vi "quiz3_vale.vi"() -> ()   [LabVIEW 2017]
panel:
  out "Usuarios Existentes 2":string[][](array[string])
  out "Leer 2":string[][](array[string])
  out "array 2":string[][](array[string])
  out "Tamaño users 2":i32
  out "Tab Control 2":enum32{"Page 1", "Page 2", "Page 3"}(tab)
  in  "Ingresar 2":bool
  in  "Usuario 2":string
  in  "Contraseña  2":string
  in  "Regresar 3":bool
  in  "ver usuarios 2":bool
  in  "Borrar usuario 2":string
  in  "Eliminar 2":bool
  in  "Agregar 2":bool
  in  "Contraseña usuario 2":string
  in  "nuevo usuario 2":string
  in  "Regresar 4":bool
  out "Leer":string[][](array[string])
  out "Usuarios Existentes":string[][](array[string])
  out "Tamaño users":i32
  out "array":string[][](array[string])
  out "Tab Control":enum32{"Page 1", "Page 2", "Page 3"}(tab)
  in  "Ingresar":bool
  in  "Usuario":string
  in  "Contraseña":string
  in  "Regresar":bool
  in  "ver usuarios":bool
  in  "Borrar usuario":string
  in  "Eliminar":bool
  in  "Agregar":bool
  in  "Contraseña usuario":string
  in  "nuevo usuario":string
  in  "Regresar 2":bool
  # "HOLIII..!"
  # "HOLIII..!"
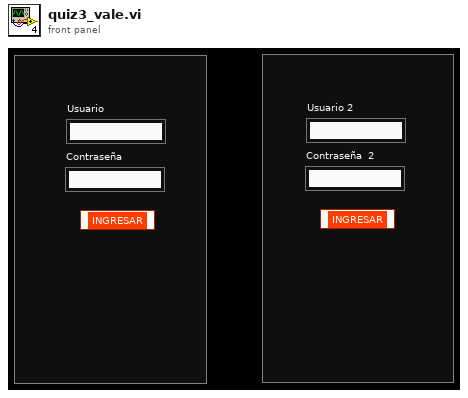
[diagram p1: front panel]
types:
  T1 = enum16{"open", "replace", "create", "open or create", "replace or create", "replace or create with confirmation"}
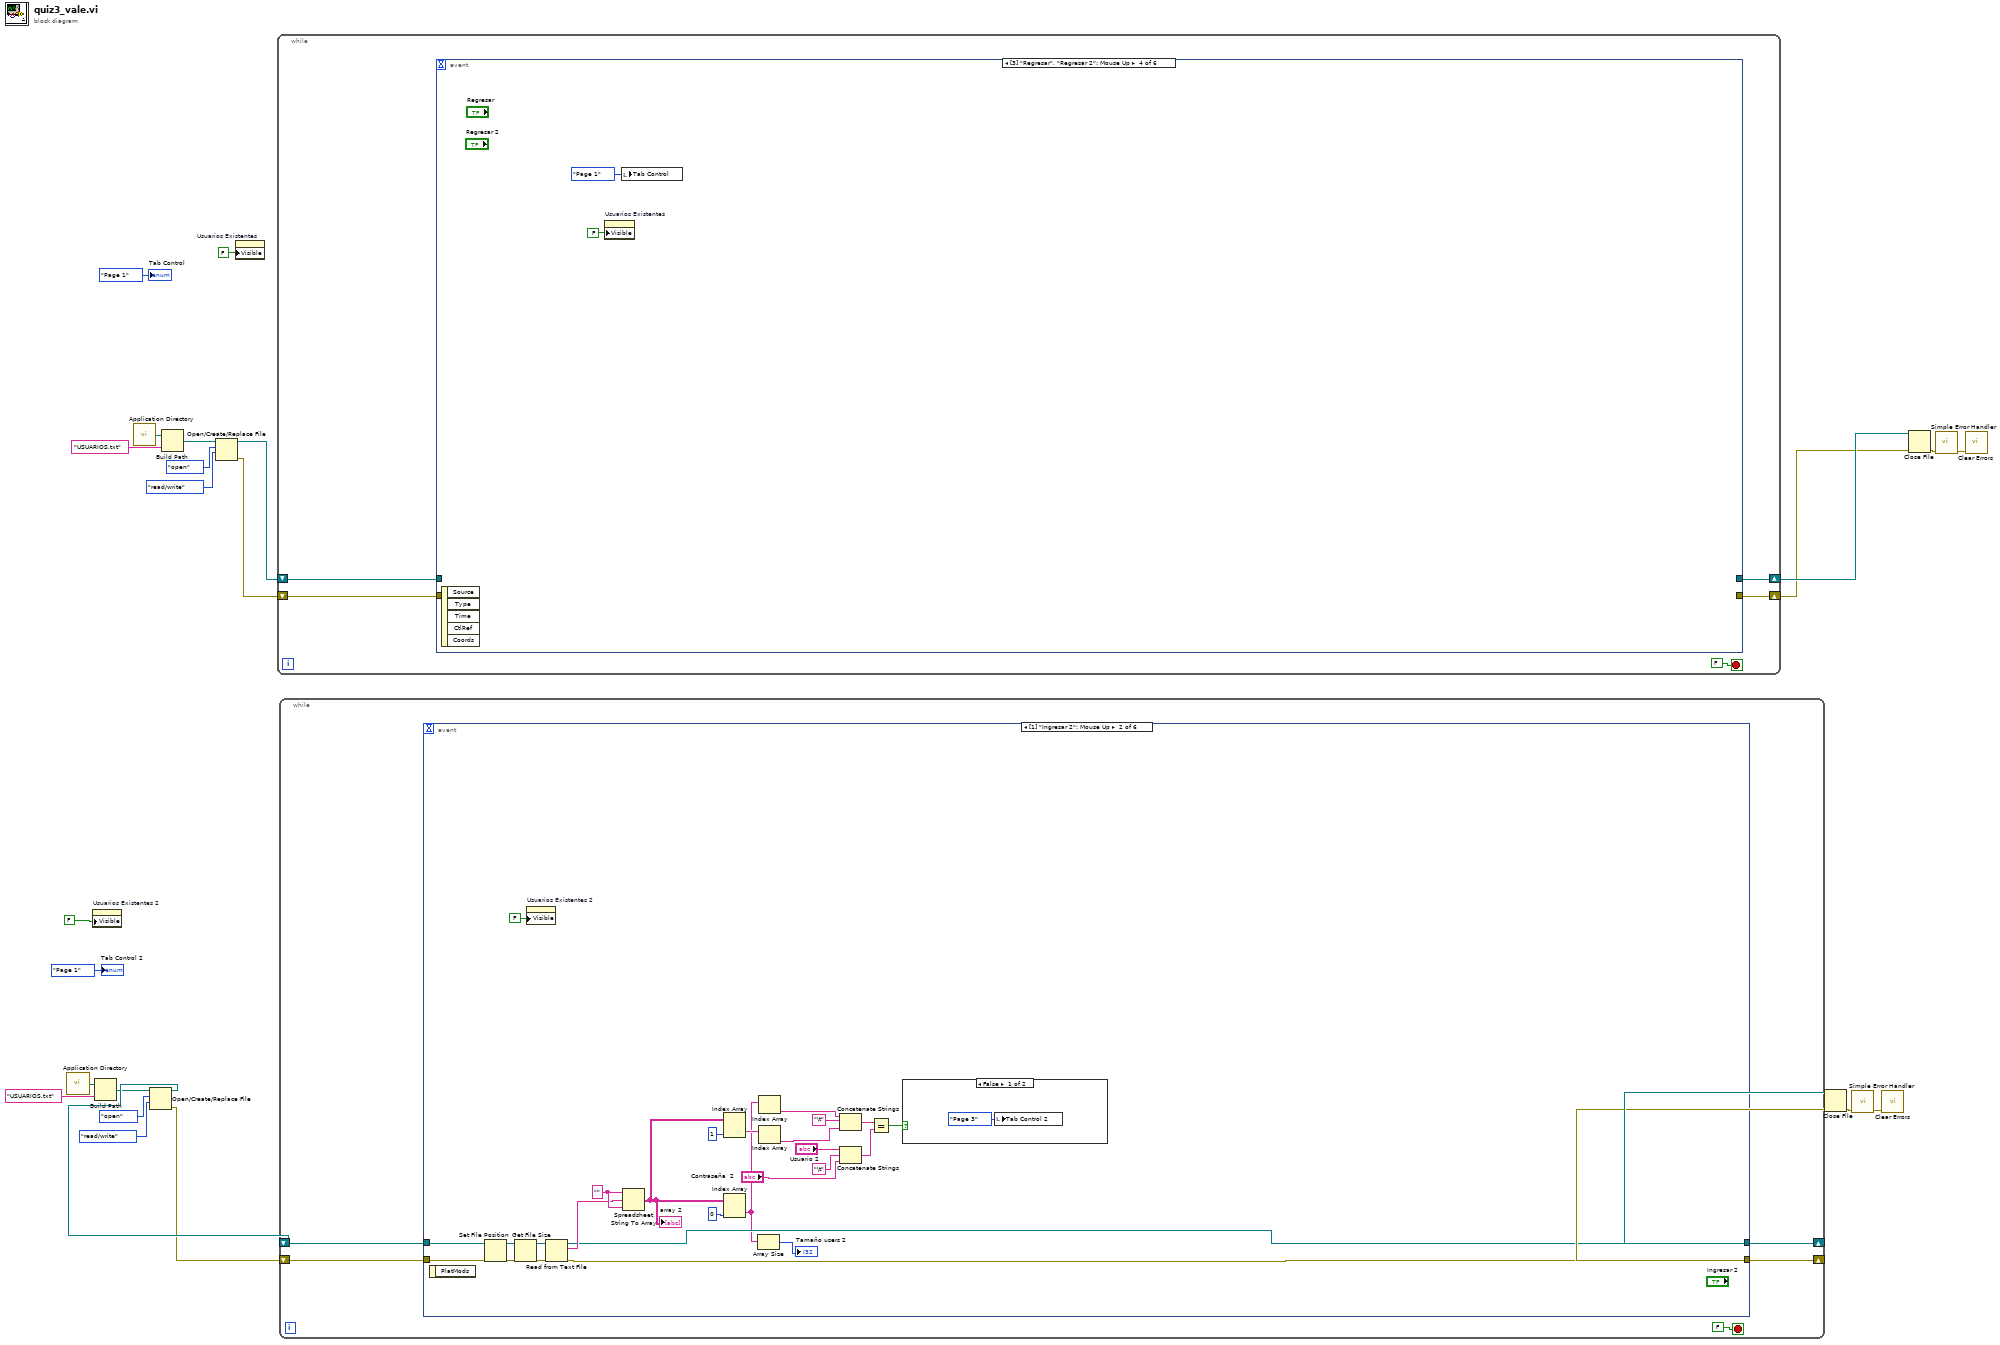
[diagram p0: block diagram]
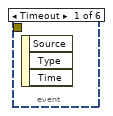
[diagram p2: hidden frame]
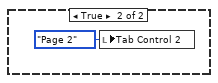
[diagram p3: hidden frame]
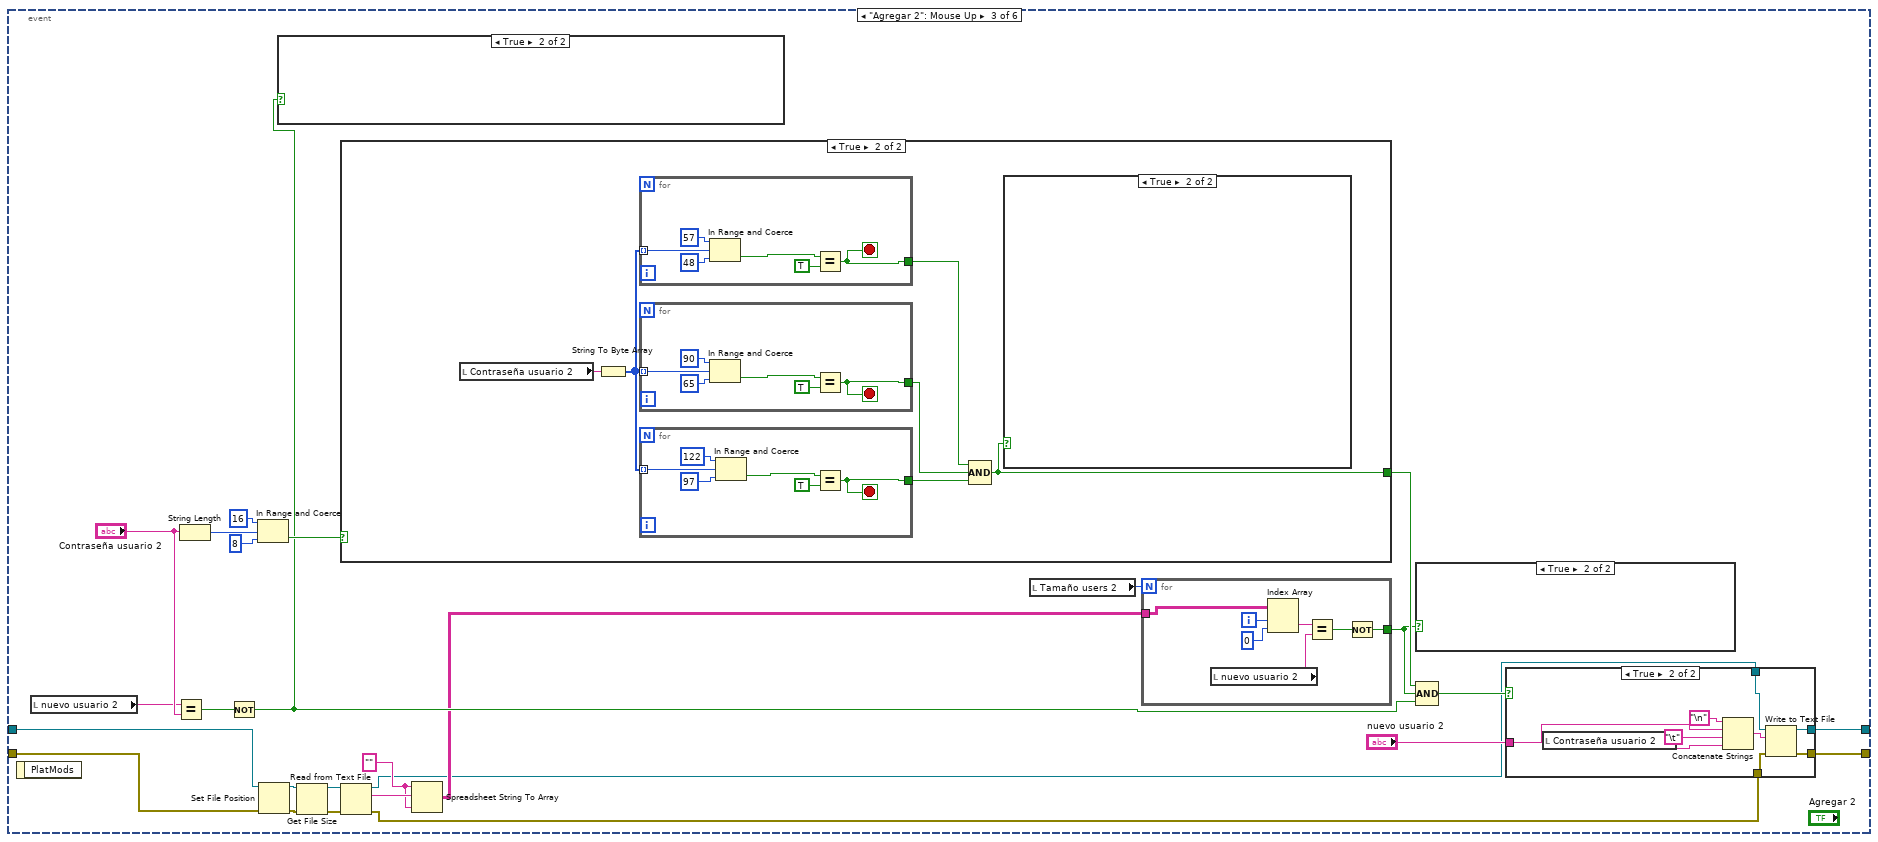
[diagram p4: hidden frame]
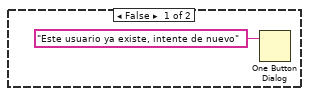
[diagram p5: hidden frame]
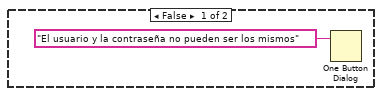
[diagram p6: hidden frame]
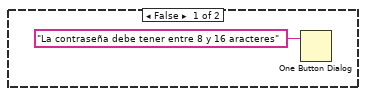
[diagram p8: hidden frame]
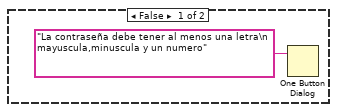
[diagram p9: hidden frame]
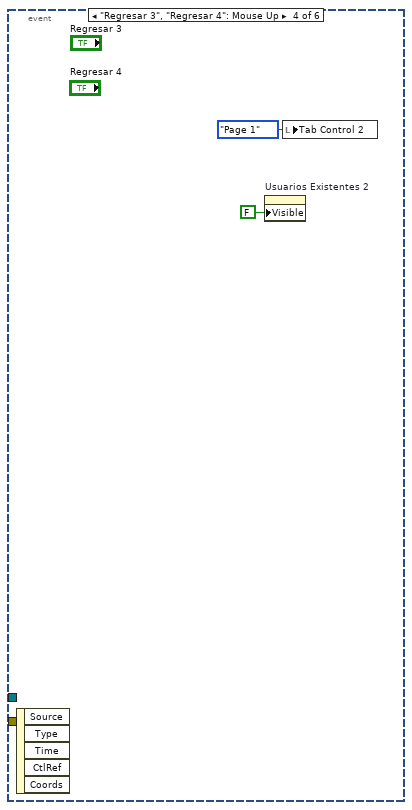
[diagram p10: hidden frame]
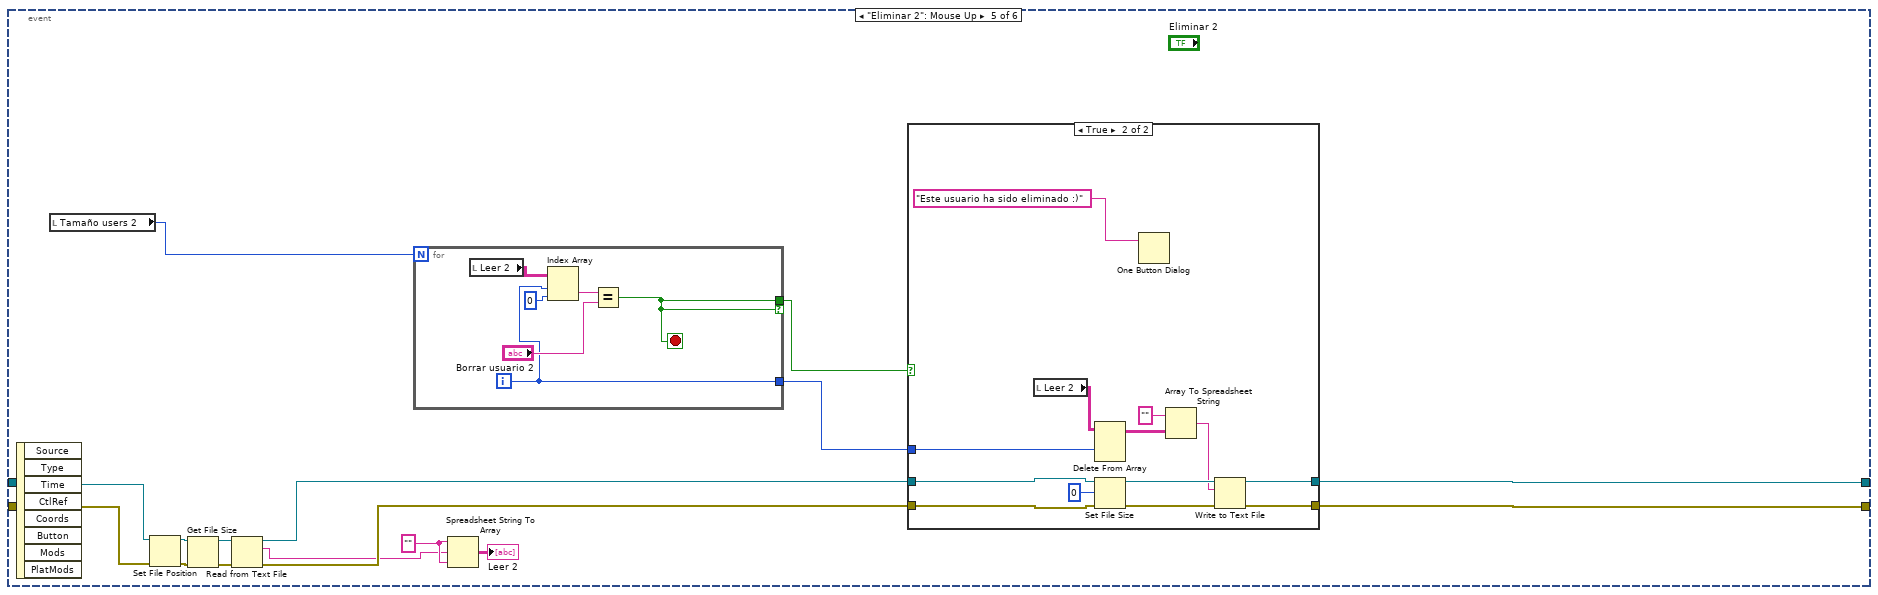
[diagram p11: hidden frame]
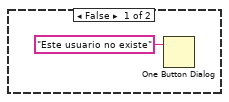
[diagram p12: hidden frame]
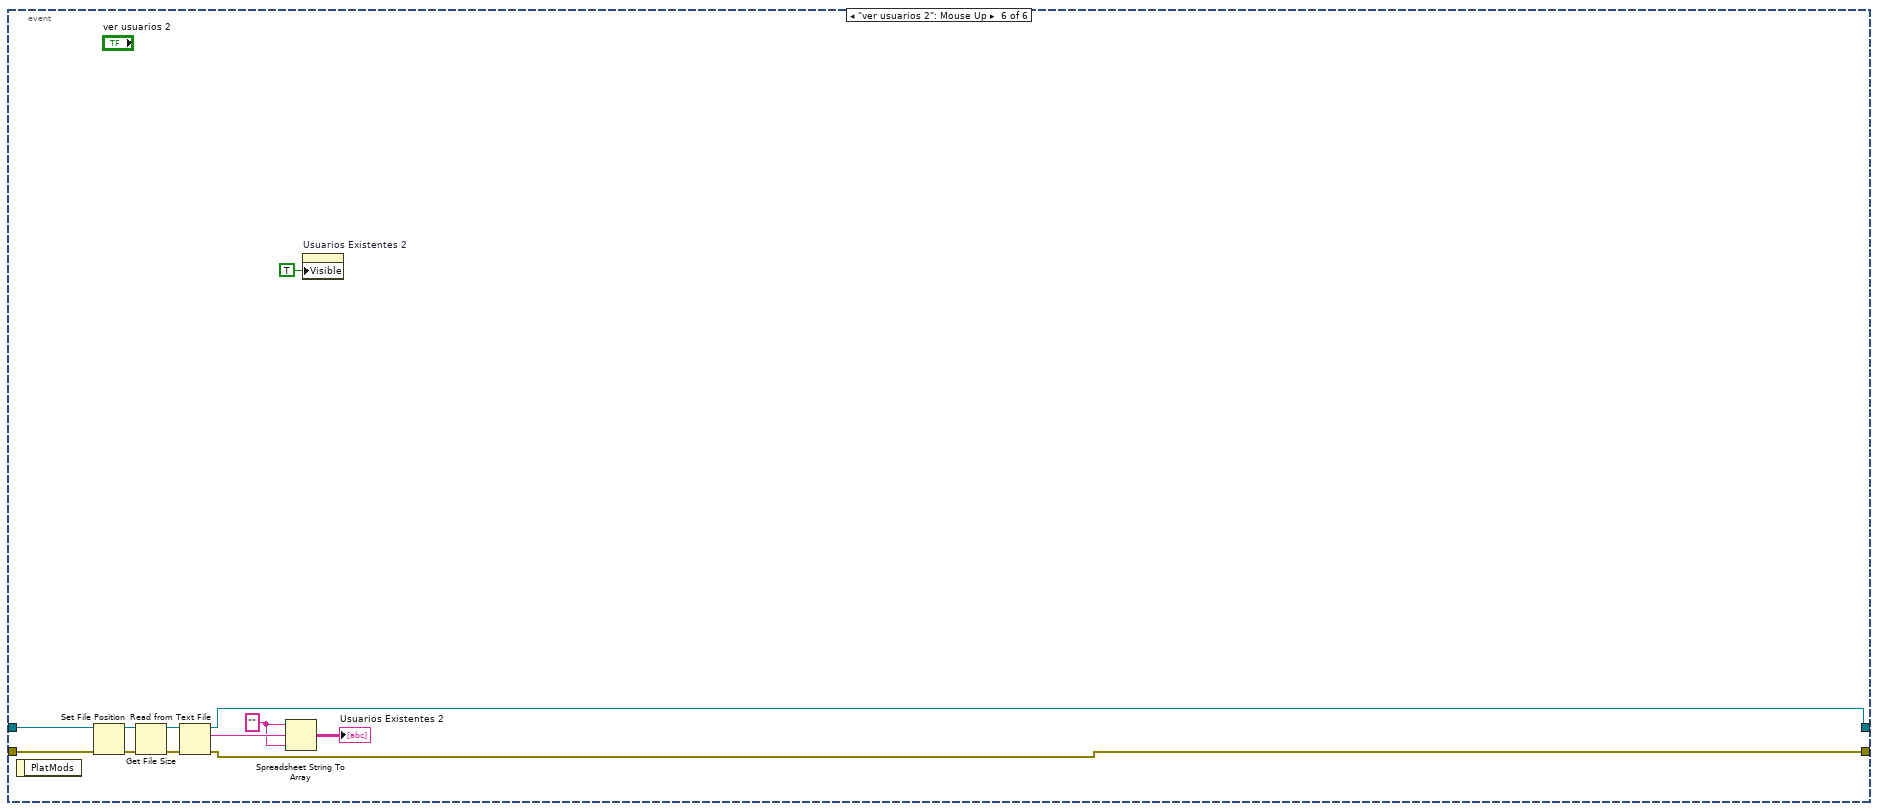
[diagram p13: hidden frame]
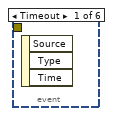
[diagram p14: hidden frame]
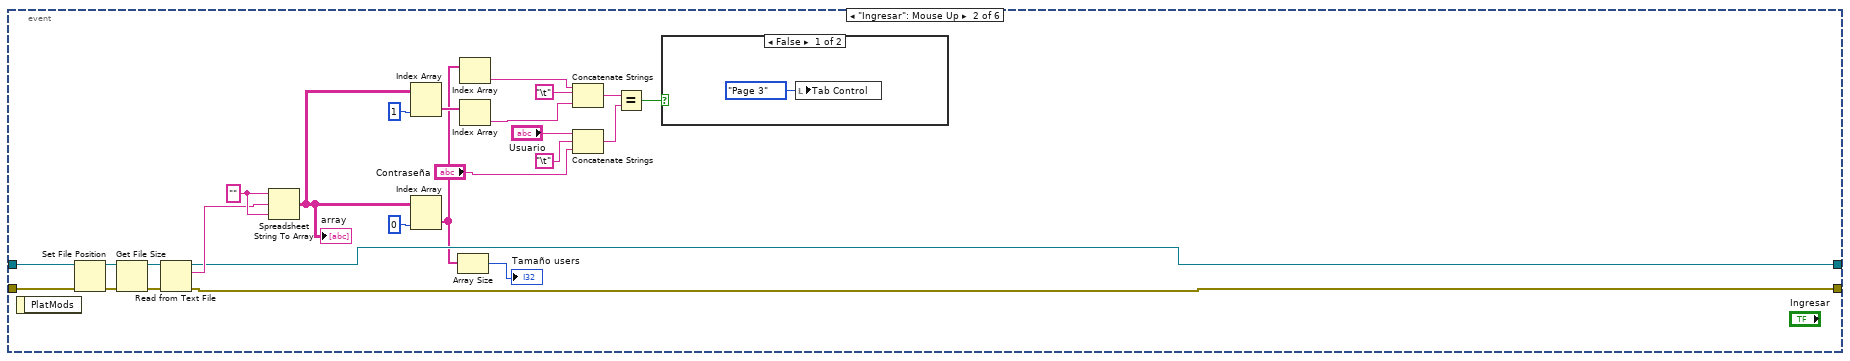
[diagram p15: hidden frame]
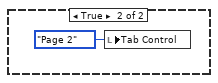
[diagram p16: hidden frame]
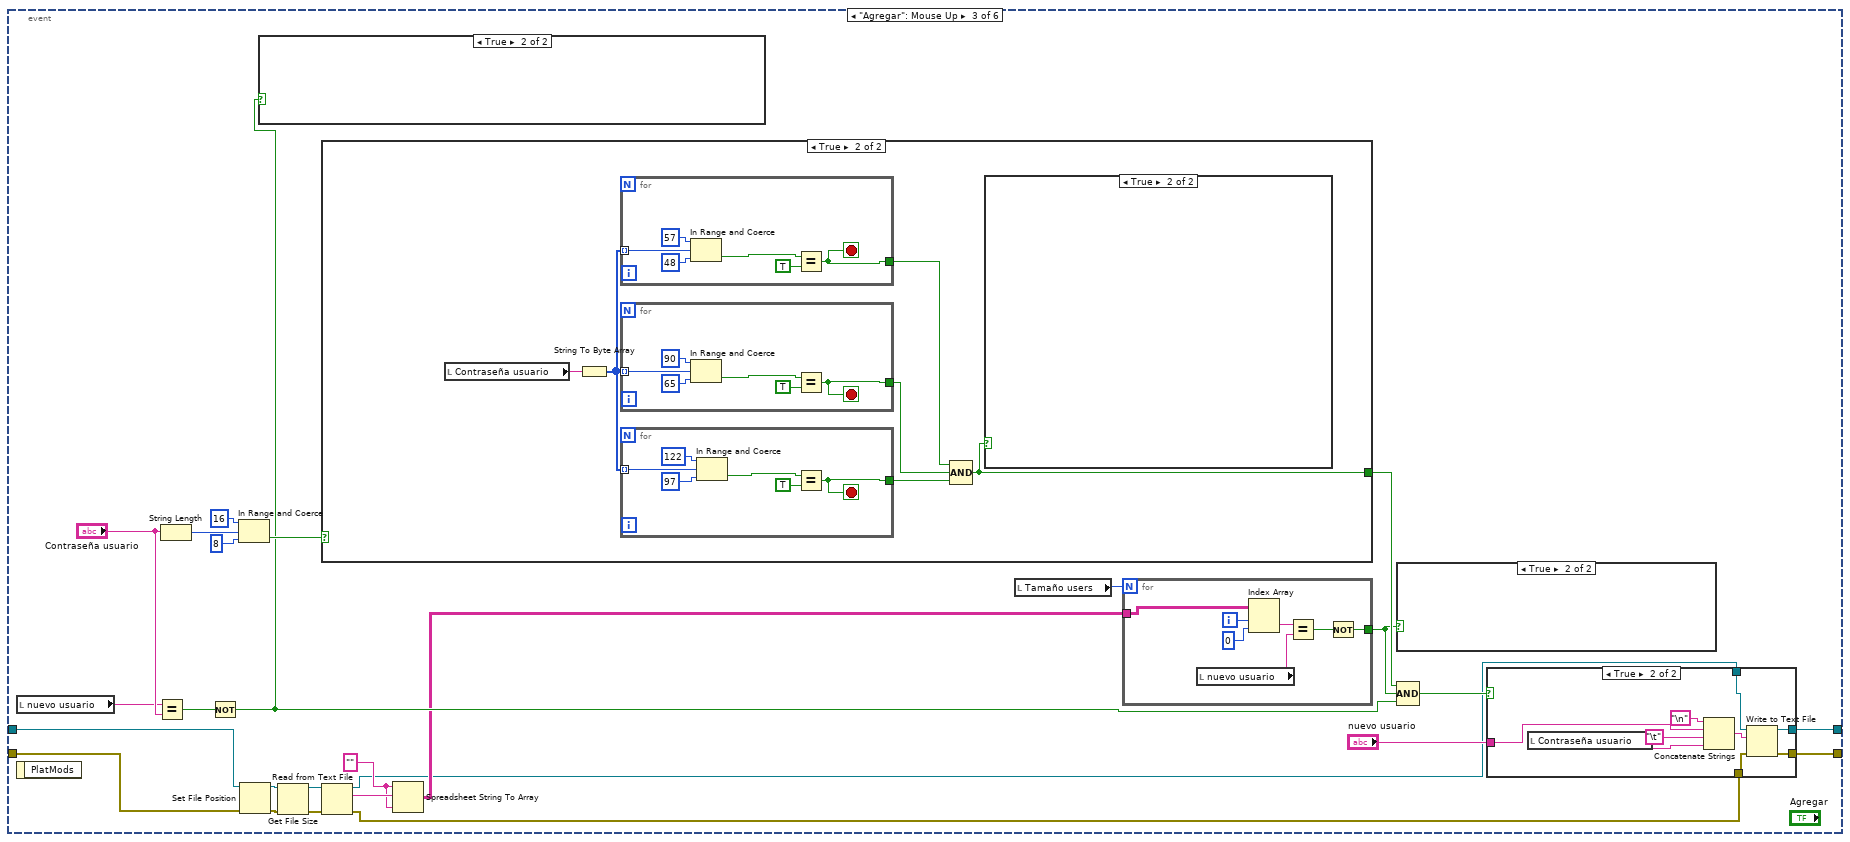
[diagram p17: hidden frame]
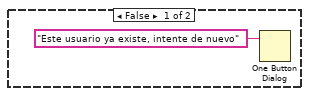
[diagram p18: hidden frame]
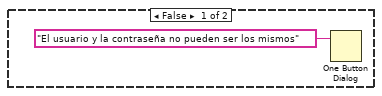
[diagram p19: hidden frame]
diagram:
  n1 = call <vilib>:"Application Directory.vi"() -> ("Application Directory"=w11:path)
  n2 = property on="Usuarios Existentes 2" class="Arr (strict)"("Visible"=FALSE) -> ()  [unwired: 2 in, 2 out]
  n3 = Build Path(base path=w11, name or relative path="USUARIOS.txt") -> (appended path=w10:path)
  n4 = call <vilib>:"Application Directory.vi"() -> ("Application Directory"=w24:path)
  n5 = Open/Create/Replace File(file path (use dialog)=w10, operation (0:open)=T1."open", access (0:read/write)=enum16{"read/write", "read-only", "write-only"}."read/write") -> (refnum out=w14:refnum<file>, error out=w13:errorcluster)  [unwired: 3 in, 1 out]
  n6 = Build Path(base path=w24, name or relative path="USUARIOS.txt") -> (appended path=w23:path)
  n7 = Open/Create/Replace File(file path (use dialog)=w23, operation (0:open)=T1."open", access (0:read/write)=enum16{"read/write", "read-only", "write-only"}."read/write") -> (refnum out=w26:refnum<file>, error out=w1:errorcluster)  [unwired: 3 in, 1 out]
  n8 = property on="Usuarios Existentes" class="Arr (strict)"("Visible"=FALSE) -> ()  [unwired: 2 in, 2 out]
  n9 = while {
    shift-right: [w28] -> w20
    shift-left: w26 -> [w30]
    shift-right: [w29] -> w19
    shift-left: w1 -> [w27]
    stop <- FALSE stop-if-true
    n10 = event shown="[3] \"Regresar\", \"Regresar 2\": Mouse Up" {
      selector: _ -> [_ _ _ _ _ _]
      dyn-events: _ -> [_ _ _ _ _ _]
      timeout: _ -> [_ _ _ _ _ _]
      tunnel: w27 -> [_ w56 w65 _ w136 w171]
      tunnel: w30 -> [_ w53 w64 _ w137 w172]
      tunnel: [_ w42 w78 _ w142 w166] -> w28
      tunnel: [_ w41 w79 _ w143 w167] -> w29
      event Timeout {
        n11 = event-data() -> ()  [unwired: 1 in, 3 out]
      }
      event "Ingresar": Mouse Up {
        w45 = "" ("format string")
        n12 = event-data() -> ()  [unwired: 1 in, 1 out]
        n13 = Set File Position(refnum=w53, error in=w56) -> (refnum out=w52:refnum<file>, error out=w55:errorcluster)  [unwired: 2 in]
        n14 = Get File Size(file=w52, error in=w55) -> (refnum out=w51:refnum<file>, 0:w54:errorcluster)  [unwired: 1 out]
        n15 = Read from Text File(file (use dialog)=w51, error in=w54) -> (refnum out=w42:refnum<file>, text=w44:string, error out=w41:errorcluster)  [unwired: 2 in, 1 out]
        n16 = Spreadsheet String To Array(format string=w45, spreadsheet string=w44, array type (2D Dbl)=w45) -> (array=w38:string[][])  [unwired: 1 in]
        "array" <- w38
        n17 = Index Array(array=w38, index (col)=1 ("disabled index (col)")) -> (element=w43:string[])  [unwired: 1 in]
        n18 = Index Array(array=w38, index (col)=0 ("disabled index (col)")) -> (element=w37:string[])  [unwired: 1 in]
        n19 = Array Size(array=w37) -> (size(s)=→"Tamaño users":i32)
        n20 = Index Array(array=w37) -> (element=w32:string)  [unwired: 1 in]
        n21 = Index Array(array=w43) -> (element=w33:string)  [unwired: 1 in]
        n22 = Concatenate Strings(w32, "\t", w33) -> (w40:string)
        n23 = Concatenate Strings("Usuario", "\t", "Contraseña") -> (w39:string)
        n24 = Equal?(x=w40, y=w39) -> (x = y?=w35:bool)
        n25 = case shown="False" w35 {
          frame False {
            n26 = local write "Tab Control"(enum32{"Page 1", "Page 2", "Page 3"}."Page 3" ("Tab Control")) -> ()
          }
          frame True {
            n27 = local write "Tab Control"(enum32{"Page 1", "Page 2", "Page 3"}."Page 2" ("Tab Control")) -> ()
          }
        }
      }
      event "Agregar": Mouse Up {
        w62 = "" ("format string")
        n28 = local read "nuevo usuario"() -> (w72:string)
        n29 = event-data() -> ()  [unwired: 1 in, 1 out]
        n30 = Equal?(x=w72, y="Contraseña usuario") -> (x = y?=w74:bool)
        n31 = String Length(string="Contraseña usuario") -> (length=w84:i32)
        n32 = Not(x=w74) -> (.not. x?=w73:bool)
        n33 = In Range and Coerce(upper limit=16, x=w84, lower limit=8) -> (In Range?=w81:bool)  [unwired: 1 out]
        n34 = Set File Position(refnum=w64, error in=w65) -> (refnum out=w68:refnum<file>, error out=w66:errorcluster)  [unwired: 2 in]
        n35 = case shown="True" w73 {
          frame False {
            n36 = One Button Dialog(message="El usuario y la contraseña no pueden ser los mismos") -> ()  [unwired: 1 in, 1 out]
          }
          frame True {
          }
        }
        n37 = Get File Size(file=w68, error in=w66) -> (refnum out=w69:refnum<file>, 0:w67:errorcluster)  [unwired: 1 out]
        n38 = case shown="True" w81 {
          tunnel: [_ w104] -> w75
          frame False {
            n39 = One Button Dialog(message="La contraseña debe tener entre 8 y 16 aracteres") -> ()  [unwired: 1 in, 1 out]
          }
          frame True {
            n40 = local read "Contraseña usuario"() -> (w109:string)
            n41 = String To Byte Array(string=w109) -> (unsigned byte array=w107:u8[])
            n42 = for {
              tunnel: w107 -> [w117] mode=indexing
              tunnel: [w116] -> w108
              stop <- w116 stop-if-true
              n43 = In Range and Coerce(upper limit=u8 57, x=w117, lower limit=u8 48) -> (In Range?=w119:bool)  [unwired: 1 out]
              n44 = Equal?(x=w119, y=TRUE) -> (x = y?=w116:bool)
            }
            n45 = for {
              tunnel: w107 -> [w113] mode=indexing
              tunnel: [w110] -> w106
              stop <- w110 stop-if-true
              n46 = In Range and Coerce(upper limit=u8 90, x=w113, lower limit=u8 65) -> (In Range?=w112:bool)  [unwired: 1 out]
              n47 = Equal?(x=w112, y=TRUE) -> (x = y?=w110:bool)
            }
            n48 = for {
              tunnel: w107 -> [w123] mode=indexing
              tunnel: [w124] -> w105
              stop <- w124 stop-if-true
              n49 = In Range and Coerce(upper limit=u8 122, x=w123, lower limit=u8 97) -> (In Range?=w126:bool)  [unwired: 1 out]
              n50 = Equal?(x=w126, y=TRUE) -> (x = y?=w124:bool)
            }
            n51 = Compound Arithmetic op=AND(w108, w106, w105) -> (w104:bool)
            n52 = case shown="True" w104 {
              frame False {
                n53 = One Button Dialog(message="La contraseña debe tener al menos una letra\n mayuscula,minuscula y un numero") -> ()  [unwired: 1 in, 1 out]
              }
              frame True {
              }
            }
          }
        }
        n54 = Read from Text File(file (use dialog)=w69, error in=w67) -> (refnum out=w59:refnum<file>, text=w63:string, error out=w60:errorcluster)  [unwired: 2 in, 1 out]
        n55 = Spreadsheet String To Array(format string=w62, spreadsheet string=w63, array type (2D Dbl)=w62) -> (array=w61:string[][])  [unwired: 1 in]
        n56 = local read "Tamaño users"() -> (w80:i32)
        n57 = for {
          N: w80 -> [_]
          tunnel: [w88] -> w70
          tunnel: w61 -> [w87]
          i -> [w92]
          n58 = local read "nuevo usuario"() -> (w90:string)
          n59 = Index Array(array=w87, index (row)=w92, index (col)=0 ("disabled index (col)")) -> (element=w91:string)
          n60 = Equal?(x=w91, y=w90) -> (x = y?=w89:bool)
          n61 = Not(x=w89) -> (.not. x?=w88:bool)
        }
        n62 = case shown="True" w70 {
          frame False {
            n63 = One Button Dialog(message="Este usuario ya existe, intente de nuevo") -> ()  [unwired: 1 in, 1 out]
          }
          frame True {
          }
        }
        n64 = Compound Arithmetic op=AND(w75, w70, w73) -> (w76:bool)
        n65 = case shown="True" w76 {
          tunnel: [_ w98] -> w78
          tunnel: [_ w97] -> w79
          tunnel: "nuevo usuario" -> [_ w96]
          tunnel: w59 -> [_ w95]
          tunnel: w60 -> [_ w94]
          frame False {
          }
          frame True {
            n66 = local read "Contraseña usuario"() -> (w99:string)
            n67 = Concatenate Strings("\n", w96, "\t", w99) -> (w100:string)
            n68 = Write to Text File(file (use dialog)=w95, text=w100, error in=w94) -> (refnum out=w98:refnum<file>, error out=w97:errorcluster)  [unwired: 1 in, 1 out]
          }
        }
      }
      event "Regresar", "Regresar 2": Mouse Up {
        n69 = event-data() -> ()  [unwired: 1 in, 5 out]
        n70 = property on="Usuarios Existentes" class="Arr (strict)"("Visible"=FALSE) -> ()  [unwired: 2 in, 2 out]
        n71 = local write "Tab Control"(enum32{"Page 1", "Page 2", "Page 3"}."Page 1" ("Tab Control")) -> ()
      }
      event "Eliminar": Mouse Up {
        w134 = "" ("format string")
        n72 = event-data() -> ()  [unwired: 1 in, 1 out]
        n73 = local read "Tamaño users"() -> (w145:i32)
        n74 = Set File Position(refnum=w137, error in=w136) -> (refnum out=w140:refnum<file>, error out=w138:errorcluster)  [unwired: 2 in]
        n75 = Get File Size(file=w140, error in=w138) -> (refnum out=w141:refnum<file>, 0:w139:errorcluster)  [unwired: 1 out]
        n76 = Read from Text File(file (use dialog)=w141, error in=w139) -> (refnum out=w135:refnum<file>, text=w133:string)  [unwired: 2 in, 2 out]
        n77 = for {
          N: w145 -> [_]
          tunnel: [w162] -> w144
          tunnel: [w159] -> w131 if=w159
          i -> [w162]
          stop <- w159 stop-if-true
          n78 = local read "Leer"() -> (w161:string[][])
          n79 = Index Array "Index Array"(array=w161, index (row)=w162, index (col)=0 ("disabled index (col)")) -> (element=w160:string)
          n80 = Equal?(x=w160, y="Borrar usuario") -> (x = y?=w159:bool)
        }
        n81 = Spreadsheet String To Array(format string=w134, spreadsheet string=w133, array type (2D Dbl)=w134) -> (array=→"Leer":string[][])  [unwired: 1 in]
        n82 = case shown="True" w131 {
          tunnel: w144 -> [_ w158]
          tunnel: w135 -> [_ w154]
          tunnel: [_ w152] -> w143
          tunnel: [_ w151] -> w142
          frame False {
            n83 = One Button Dialog(message="Este usuario no existe") -> ()  [unwired: 1 in, 1 out]
          }
          frame True {
            n84 = local read "Leer"() -> (w149:string[][])
            n85 = Delete From Array "Delete From Array"(array=w149, index (row)=w158) -> (array with subset deleted=w148:string[][])  [unwired: 2 in, 1 out]
            n86 = Set File Size(6:i64 0 ("size (in bytes)"), 7:w154) -> (0:w153:errorcluster, 3:w156:refnum<file>)  [unwired: 1 in]
            n87 = One Button Dialog(message="Este usuario ha sido eliminado :)") -> ()  [unwired: 1 in, 1 out]
            n88 = Array To Spreadsheet String(array=w148, 3:"" ("format string")) -> (spreadsheet string=w155:string)  [unwired: 1 in]
            n89 = Write to Text File(file (use dialog)=w156, text=w155, error in=w153) -> (refnum out=w151:refnum<file>, error out=w152:errorcluster)  [unwired: 1 in, 1 out]
          }
        }
      }
      event "ver usuarios": Mouse Up {
        w169 = "" ("format string")
        n90 = event-data() -> ()  [unwired: 1 in, 1 out]
        n91 = Set File Position(refnum=w172, error in=w171) -> (refnum out=w175:refnum<file>, error out=w173:errorcluster)  [unwired: 2 in]
        n92 = Get File Size(file=w175, error in=w173) -> (refnum out=w176:refnum<file>, 0:w174:errorcluster)  [unwired: 1 out]
        n93 = Read from Text File(file (use dialog)=w176, error in=w174) -> (refnum out=w166:refnum<file>, text=w170:string, error out=w167:errorcluster)  [unwired: 2 in, 1 out]
        n94 = Spreadsheet String To Array(format string=w169, spreadsheet string=w170, array type (2D Dbl)=w169) -> (array=→"Usuarios Existentes":string[][])  [unwired: 1 in]
        n95 = property on="Usuarios Existentes" class="Arr (strict)"("Visible"=TRUE) -> ()  [unwired: 2 in, 2 out]
      }
    }
  }
  n96 = while {
    shift-right: [w178] -> w7
    shift-left: w14 -> [w180]
    shift-right: [w179] -> w6
    shift-left: w13 -> [w177]
    stop <- FALSE stop-if-true
    n97 = event shown="[1] \"Ingresar 2\": Mouse Up" {
      selector: _ -> [_ _ _ _ _ _]
      dyn-events: _ -> [_ _ _ _ _ _]
      timeout: _ -> [_ _ _ _ _ _]
      tunnel: w177 -> [_ w207 w216 _ w288 w324]
      tunnel: w180 -> [_ w204 w215 _ w289 w325]
      tunnel: [_ w193 w229 _ w294 w319] -> w178
      tunnel: [_ w192 w230 _ w295 w320] -> w179
      event Timeout {
        n98 = event-data() -> ()  [unwired: 1 in, 3 out]
      }
      event "Ingresar 2": Mouse Up {
        w196 = "" ("format string")
        n99 = event-data() -> ()  [unwired: 1 in, 1 out]
        n100 = Set File Position(refnum=w204, error in=w207) -> (refnum out=w203:refnum<file>, error out=w206:errorcluster)  [unwired: 2 in]
        n101 = Get File Size(file=w203, error in=w206) -> (refnum out=w202:refnum<file>, 0:w205:errorcluster)  [unwired: 1 out]
        n102 = property on="Usuarios Existentes 2" class="Arr (strict)"("Visible"=FALSE) -> ()  [unwired: 2 in, 2 out]
        n103 = Read from Text File(file (use dialog)=w202, error in=w205) -> (refnum out=w193:refnum<file>, text=w195:string, error out=w192:errorcluster)  [unwired: 2 in, 1 out]
        n104 = Spreadsheet String To Array(format string=w196, spreadsheet string=w195, array type (2D Dbl)=w196) -> (array=w189:string[][])  [unwired: 1 in]
        "array 2" <- w189
        n105 = Index Array(array=w189, index (col)=1 ("disabled index (col)")) -> (element=w194:string[])  [unwired: 1 in]
        n106 = Index Array(array=w189, index (col)=0 ("disabled index (col)")) -> (element=w188:string[])  [unwired: 1 in]
        n107 = Array Size(array=w188) -> (size(s)=→"Tamaño users 2":i32)
        n108 = Index Array(array=w188) -> (element=w183:string)  [unwired: 1 in]
        n109 = Index Array(array=w194) -> (element=w184:string)  [unwired: 1 in]
        n110 = Concatenate Strings(w183, "\t", w184) -> (w191:string)
        n111 = Concatenate Strings("Usuario 2", "\t", "Contraseña  2") -> (w190:string)
        n112 = Equal?(x=w191, y=w190) -> (x = y?=w186:bool)
        n113 = case shown="False" w186 {
          frame False {
            n114 = local write "Tab Control 2"(enum32{"Page 1", "Page 2", "Page 3"}."Page 3" ("Tab Control")) -> ()
          }
          frame True {
            n115 = local write "Tab Control 2"(enum32{"Page 1", "Page 2", "Page 3"}."Page 2" ("Tab Control")) -> ()
          }
        }
      }
      event "Agregar 2": Mouse Up {
        w213 = "" ("format string")
        n116 = event-data() -> ()  [unwired: 1 in, 1 out]
        n117 = local read "nuevo usuario 2"() -> (w223:string)
        n118 = Equal?(x=w223, y="Contraseña usuario 2") -> (x = y?=w225:bool)
        n119 = String Length(string="Contraseña usuario 2") -> (length=w235:i32)
        n120 = Not(x=w225) -> (.not. x?=w224:bool)
        n121 = In Range and Coerce(upper limit=16, x=w235, lower limit=8) -> (In Range?=w232:bool)  [unwired: 1 out]
        n122 = Set File Position(refnum=w215, error in=w216) -> (refnum out=w219:refnum<file>, error out=w217:errorcluster)  [unwired: 2 in]
        n123 = case shown="True" w224 {
          frame False {
            n124 = One Button Dialog(message="El usuario y la contraseña no pueden ser los mismos") -> ()  [unwired: 1 in, 1 out]
          }
          frame True {
          }
        }
        n125 = Get File Size(file=w219, error in=w217) -> (refnum out=w220:refnum<file>, 0:w218:errorcluster)  [unwired: 1 out]
        n126 = case shown="True" w232 {
          tunnel: [_ w255] -> w226
          frame False {
            n127 = One Button Dialog(message="La contraseña debe tener entre 8 y 16 aracteres") -> ()  [unwired: 1 in, 1 out]
          }
          frame True {
            n128 = local read "Contraseña usuario 2"() -> (w260:string)
            n129 = String To Byte Array(string=w260) -> (unsigned byte array=w258:u8[])
            n130 = for {
              tunnel: w258 -> [w268] mode=indexing
              tunnel: [w267] -> w259
              stop <- w267 stop-if-true
              n131 = In Range and Coerce(upper limit=u8 57, x=w268, lower limit=u8 48) -> (In Range?=w270:bool)  [unwired: 1 out]
              n132 = Equal?(x=w270, y=TRUE) -> (x = y?=w267:bool)
            }
            n133 = for {
              tunnel: w258 -> [w264] mode=indexing
              tunnel: [w261] -> w257
              stop <- w261 stop-if-true
              n134 = In Range and Coerce(upper limit=u8 90, x=w264, lower limit=u8 65) -> (In Range?=w263:bool)  [unwired: 1 out]
              n135 = Equal?(x=w263, y=TRUE) -> (x = y?=w261:bool)
            }
            n136 = for {
              tunnel: w258 -> [w274] mode=indexing
              tunnel: [w275] -> w256
              stop <- w275 stop-if-true
              n137 = In Range and Coerce(upper limit=u8 122, x=w274, lower limit=u8 97) -> (In Range?=w277:bool)  [unwired: 1 out]
              n138 = Equal?(x=w277, y=TRUE) -> (x = y?=w275:bool)
            }
            n139 = Compound Arithmetic op=AND(w259, w257, w256) -> (w255:bool)
            n140 = case shown="True" w255 {
              frame False {
                n141 = One Button Dialog(message="La contraseña debe tener al menos una letra\n mayuscula,minuscula y un numero") -> ()  [unwired: 1 in, 1 out]
              }
              frame True {
              }
            }
          }
        }
        n142 = Read from Text File(file (use dialog)=w220, error in=w218) -> (refnum out=w210:refnum<file>, text=w214:string, error out=w211:errorcluster)  [unwired: 2 in, 1 out]
        n143 = Spreadsheet String To Array(format string=w213, spreadsheet string=w214, array type (2D Dbl)=w213) -> (array=w212:string[][])  [unwired: 1 in]
        n144 = local read "Tamaño users 2"() -> (w231:i32)
        n145 = for {
          N: w231 -> [_]
          tunnel: [w239] -> w221
          tunnel: w212 -> [w238]
          i -> [w243]
          n146 = local read "nuevo usuario 2"() -> (w241:string)
          n147 = Index Array(array=w238, index (row)=w243, index (col)=0 ("disabled index (col)")) -> (element=w242:string)
          n148 = Equal?(x=w242, y=w241) -> (x = y?=w240:bool)
          n149 = Not(x=w240) -> (.not. x?=w239:bool)
        }
        n150 = case shown="True" w221 {
          frame False {
            n151 = One Button Dialog(message="Este usuario ya existe, intente de nuevo") -> ()  [unwired: 1 in, 1 out]
          }
          frame True {
          }
        }
        n152 = Compound Arithmetic op=AND(w226, w221, w224) -> (w227:bool)
        n153 = case shown="True" w227 {
          tunnel: [_ w249] -> w229
          tunnel: [_ w248] -> w230
          tunnel: "nuevo usuario 2" -> [_ w247]
          tunnel: w210 -> [_ w246]
          tunnel: w211 -> [_ w245]
          frame False {
          }
          frame True {
            n154 = local read "Contraseña usuario 2"() -> (w250:string)
            n155 = Concatenate Strings("\n", w247, "\t", w250) -> (w251:string)
            n156 = Write to Text File(file (use dialog)=w246, text=w251, error in=w245) -> (refnum out=w249:refnum<file>, error out=w248:errorcluster)  [unwired: 1 in, 1 out]
          }
        }
      }
      event "Regresar 3", "Regresar 4": Mouse Up {
        n157 = event-data() -> ()  [unwired: 1 in, 5 out]
        n158 = property on="Usuarios Existentes 2" class="Arr (strict)"("Visible"=FALSE) -> ()  [unwired: 2 in, 2 out]
        n159 = local write "Tab Control 2"(enum32{"Page 1", "Page 2", "Page 3"}."Page 1" ("Tab Control")) -> ()
      }
      event "Eliminar 2": Mouse Up {
        w285 = "" ("format string")
        n160 = event-data() -> ()  [unwired: 1 in, 8 out]
        n161 = local read "Tamaño users 2"() -> (w297:i32)
        n162 = Set File Position(refnum=w289, error in=w288) -> (refnum out=w292:refnum<file>, error out=w290:errorcluster)  [unwired: 2 in]
        n163 = Get File Size(file=w292, error in=w290) -> (refnum out=w293:refnum<file>, 0:w291:errorcluster)  [unwired: 1 out]
        n164 = Read from Text File(file (use dialog)=w293, error in=w291) -> (refnum out=w287:refnum<file>, text=w284:string, error out=w286:errorcluster)  [unwired: 2 in, 1 out]
        n165 = for {
          N: w297 -> [_]
          tunnel: [w315] -> w296
          tunnel: [w312] -> w282 if=w312
          i -> [w315]
          stop <- w312 stop-if-true
          n166 = local read "Leer 2"() -> (w314:string[][])
          n167 = Index Array "Index Array"(array=w314, index (row)=w315, index (col)=0 ("disabled index (col)")) -> (element=w313:string)
          n168 = Equal?(x=w313, y="Borrar usuario 2") -> (x = y?=w312:bool)
        }
        n169 = Spreadsheet String To Array(format string=w285, spreadsheet string=w284, array type (2D Dbl)=w285) -> (array=→"Leer 2":string[][])  [unwired: 1 in]
        n170 = case shown="True" w282 {
          tunnel: w296 -> [_ w311]
          tunnel: w287 -> [_ w307]
          tunnel: w286 -> [_ w306]
          tunnel: [_ w304] -> w295
          tunnel: [_ w303] -> w294
          frame False {
            n171 = One Button Dialog(message="Este usuario no existe") -> ()  [unwired: 1 in, 1 out]
          }
          frame True {
            n172 = local read "Leer 2"() -> (w301:string[][])
            n173 = Delete From Array "Delete From Array"(array=w301, index (row)=w311) -> (array with subset deleted=w300:string[][])  [unwired: 2 in, 1 out]
            n174 = Set File Size(4:w306, 6:i64 0 ("size (in bytes)"), 7:w307) -> (0:w305:errorcluster, 3:w309:refnum<file>)
            n175 = One Button Dialog(message="Este usuario ha sido eliminado :)") -> ()  [unwired: 1 in, 1 out]
            n176 = Array To Spreadsheet String(array=w300, 3:"" ("format string")) -> (spreadsheet string=w308:string)  [unwired: 1 in]
            n177 = Write to Text File(file (use dialog)=w309, text=w308, error in=w305) -> (refnum out=w303:refnum<file>, error out=w304:errorcluster)  [unwired: 1 in, 1 out]
          }
        }
      }
      event "ver usuarios 2": Mouse Up {
        w322 = "" ("format string")
        n178 = event-data() -> ()  [unwired: 1 in, 1 out]
        n179 = Set File Position(refnum=w325, error in=w324) -> (refnum out=w328:refnum<file>, error out=w326:errorcluster)  [unwired: 2 in]
        n180 = Get File Size(file=w328, error in=w326) -> (refnum out=w329:refnum<file>, 0:w327:errorcluster)  [unwired: 1 out]
        n181 = Read from Text File(file (use dialog)=w329, error in=w327) -> (refnum out=w319:refnum<file>, text=w323:string, error out=w320:errorcluster)  [unwired: 2 in, 1 out]
        n182 = Spreadsheet String To Array(format string=w322, spreadsheet string=w323, array type (2D Dbl)=w322) -> (array=→"Usuarios Existentes 2":string[][])  [unwired: 1 in]
        n183 = property on="Usuarios Existentes 2" class="Arr (strict)"("Visible"=TRUE) -> ()  [unwired: 2 in, 2 out]
      }
    }
  }
  n184 = Close File(refnum=w7, error in=w6) -> (error out=w5:errorcluster)  [unwired: 1 out]
  n185 = call <vilib>:"Simple Error Handler.vi"("error in (no error)"=w5) -> ("error out"=w4:errorcluster)  [unwired: 4 in, 4 out]
  n186 = call <vilib>:"Clear Errors.vi"("error in (no error)"=w4) -> ()  [unwired: 5 in, 2 out]
  n187 = Close File(refnum=w20, error in=w19) -> (error out=w18:errorcluster)  [unwired: 1 out]
  n188 = call <vilib>:"Simple Error Handler.vi"("error in (no error)"=w18) -> ("error out"=w17:errorcluster)  [unwired: 4 in, 4 out]
  n189 = call <vilib>:"Clear Errors.vi"("error in (no error)"=w17) -> ()  [unwired: 5 in, 2 out]
  "Tab Control" <- enum32{"Page 1", "Page 2", "Page 3"}."Page 1" ("Tab Control")
  "Tab Control 2" <- enum32{"Page 1", "Page 2", "Page 3"}."Page 1" ("Tab Control")
